vi "kloehn V6 - Close Comm .vi"(8 "error in":errorcluster, 11 "VISA Ref":refnum<visa-resource-name>="ASRL1::INSTR") -> (0 "error out":errorcluster)   [LabVIEW 2010]
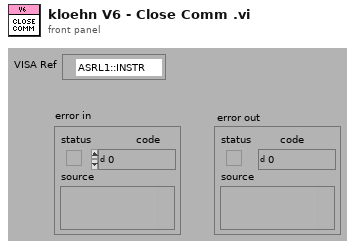
[diagram p1: front panel]
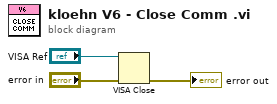
[diagram p0: block diagram]
diagram:
  n1 = VISA Close(VISA resource name="VISA Ref", error in (no error)="error in") -> (error out=→"error out":errorcluster)
